vi "Integrator Start-Stop.vi"(8 "error in (no error)":errorcluster, 9 "Start/Stop (F: Stop)":bool, 10 "Element (All: 0)":T1(ring), 11 "Yokogawa WT500 in":refnum<class "Yokogawa WT500.lvclass">) -> (0 "error out":errorcluster, 3 "Yokogawa WT500 out":refnum<class "Yokogawa WT500.lvclass">)   [LabVIEW 2016, in "Generic Power Analyzer.lvlib" / "Yokogawa WT500.lvlib" / "Yokogawa WT500.lvclass"]
uses:
  Yokogawa WT500.lvclass
  Generic Power Analyzer/Generic Power Analyzer.lvclass
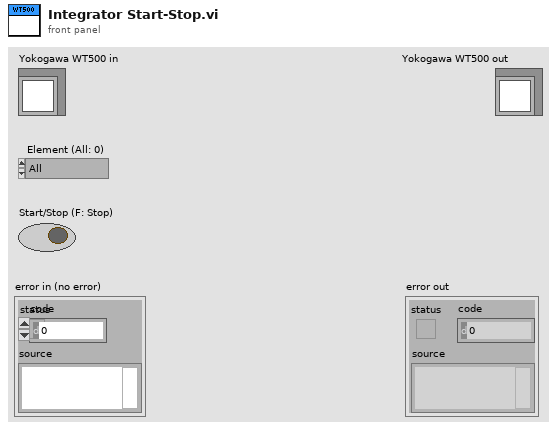
[diagram p1: front panel]
types:
  T1 = enum16{"All", "Element 1", "Element 2", "Element 3", "Element 4", "Element 5", "Element 6"}
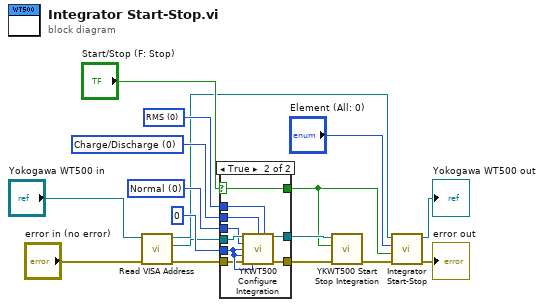
[diagram p0: block diagram]
diagram:
  w14 = u16 0 items=["Charge/Discharge", "Sold/Bought"] ("WP Type (0: Charge/Discharge)")
  w15 = u16 0 items=["RMS", "MEAN", "DC", "R-MEAN", "AC"] ("Q Mode (2: DC)")
  w17 = u16 0 items=["Normal", "Continuous", "R-Normal", "R-Continuous"] ("Integration Mode (0: Normal)")
  n1 = call-dynamic "Read VISA Address.vi"("error in (no error)"="error in (no error)", "Generic Device in"="Yokogawa WT500 in") -> ("error out"=w3:errorcluster, "VISA Address"=w2:refnum<visa-resource-name>, "Generic Device out"=w1:refnum<class "Yokogawa WT500.lvclass">)  [unwired: 7 in]
  n2 = case shown="True" "Start/Stop (F: Stop)" {
    selector: "Start/Stop (F: Stop)" -> [w18 w21]
    tunnel: w2 -> [w20 w29]
    tunnel: w17 -> [_ w28]
    tunnel: 0 ("Integration Time Hour (0)") -> [_ w27]
    tunnel: w15 -> [_ w26]
    tunnel: w14 -> [_ w25]
    tunnel: [w20 w24] -> w13
    tunnel: [w19 w23] -> w12
    tunnel: w3 -> [w19 w22]
    tunnel: [w18 w21] -> w6
    frame False {
    }
    frame True {
      n3 = call <instrlib>:"YKWT500 Configure Integration.vi"("VISA resource name"=w29, "WP Type (0: Charge/Discharge)"=w25, "Q Mode (2: DC)"=w26, "Integration Mode (0: Normal)"=w28, "Integration Time Hour (0)"=w27, "Integration Time Minute (0)"=w27, "error in (no error)"=w22, "Integration Time Second (0)"=w27) -> ("VISA resource name out"=w24:refnum<visa-resource-name>, "error out"=w23:errorcluster)  [unwired: 6 in]
    }
  }
  n4 = call <instrlib>:"YKWT500 Start Stop Integration.vi"("error in (no error)"=w12, "Start/Stop (False: Stop)"=w6, "VISA resource name"=w13) -> ("error out"=w10:errorcluster)  [unwired: 7 in, 1 out]
  n5 = call-parent "Integrator Start-Stop.vi"("error in (no error)"=w10, "Start/Stop"=w6, "Element (All: 0)"="Element (All: 0)", "Generic Power Analyzer in"=w1) -> ("error out"=→"error out":errorcluster, "Generic Power Analyzer out"=→"Yokogawa WT500 out":refnum<class "Yokogawa WT500.lvclass">)  [unwired: 6 in]
